vi "Write Max File Size.vi"(8 "error in (no error)":errorcluster, 10 "Max File Size":i64=10485760, 11 "Error in":refnum<class "Error.lvclass">) -> (0 "error out":errorcluster, 3 "Error out":refnum<class "Error.lvclass">)   [LabVIEW 2019, in "TSC Error.lvlib" / "Error.lvclass"]
uses:
  Error.lvclass
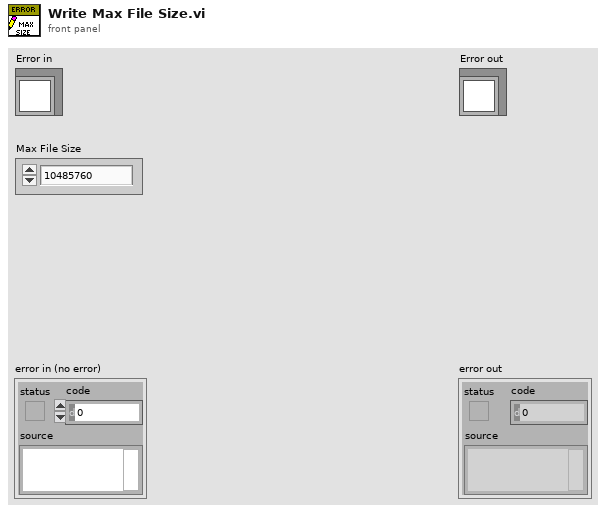
[diagram p1: front panel]
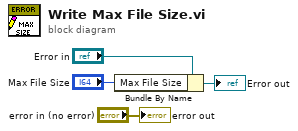
[diagram p0: block diagram]
diagram:
  n1 = Bundle By Name(cluster="Error in", "Max File Size"="Max File Size") -> (→"Error out":refnum<class "Error.lvclass">)
  "error out" <- "error in (no error)"
